vi "DISP_ENABLE.vi"(0 "VISA IN":refnum<visa-resource-name>, 5 "error in":errorcluster, 7 "ON | OFF":bool) -> (14 "VISA Out":refnum<visa-resource-name>, 19 "error out":errorcluster)   [LabVIEW 2018, in "PNA-X.lvlib"]
doc: "DISPlay:ENABLE <ON | OFF> \n(Read-Write) Specifies whether to disable or enable all analyzer display information in all windows \nin the analyzer application. Marker data is not updated. More CPU time is spent making \nmeasurements instead of updating the display. \nParameters \n<ON | OFF> ON (or 1) - turns the display ON. \nOFF (or 0) - turns the display OFF. \nExamples DISP:ENAB ON \ndisplay:enable off \nQuery Syntax DISPlay:ENABle? \nReturn Type Boolean (1 = ON, 0 = OFF) \nDefault ON"
uses:
  PNA-X.lvlib
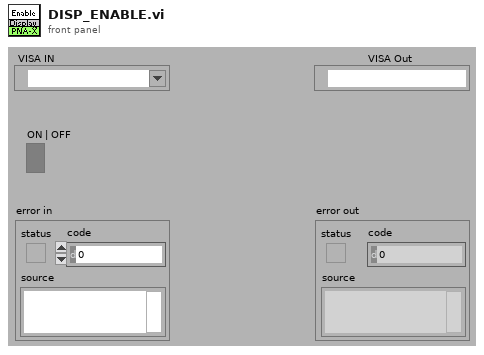
[diagram p1: front panel]
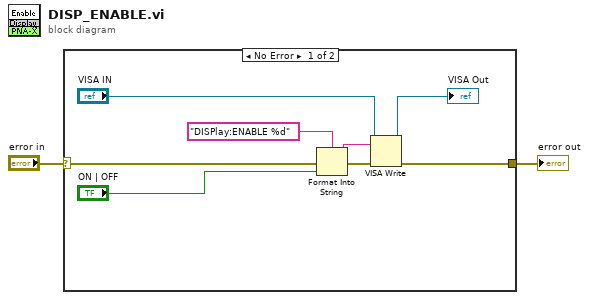
[diagram p0: block diagram]
diagram:
  n1 = case shown="No Error" "error in" {
    selector: "error in" -> [w10 w11]
    tunnel: [w5 w11] -> w1
    frame No Error {
      n2 = Format Into String(format string="DISPlay:ENABLE %d" ("Cmdline"), error in=w10, "ON | OFF") -> (resulting string=w8:string, error out=w9:errorcluster)  [unwired: 1 in]
      n3 = VISA Write(VISA resource name="VISA IN", write buffer=w8, error in (no error)=w9) -> (VISA resource name out=→"VISA Out":refnum<visa-resource-name>, error out=w5:errorcluster)  [unwired: 1 out]
    }
    frame Error {
    }
  }
  "error out" <- w1
